vi "h.ACQ.GetFullSpectrumStreamToStoragePercentComplete.vi"(8 "error in":errorcluster, 11 "Connection ID":refnum<k5>) -> (0 "error out":errorcluster, 2 "Percent Complete":i32, 3 "Connection ID out":refnum<k5>)   [LabVIEW 2016, in "h.Library.lvlib"]
uses:
  h.Library.lvlib
panel:
  out "Content":u8[](array[numeric])
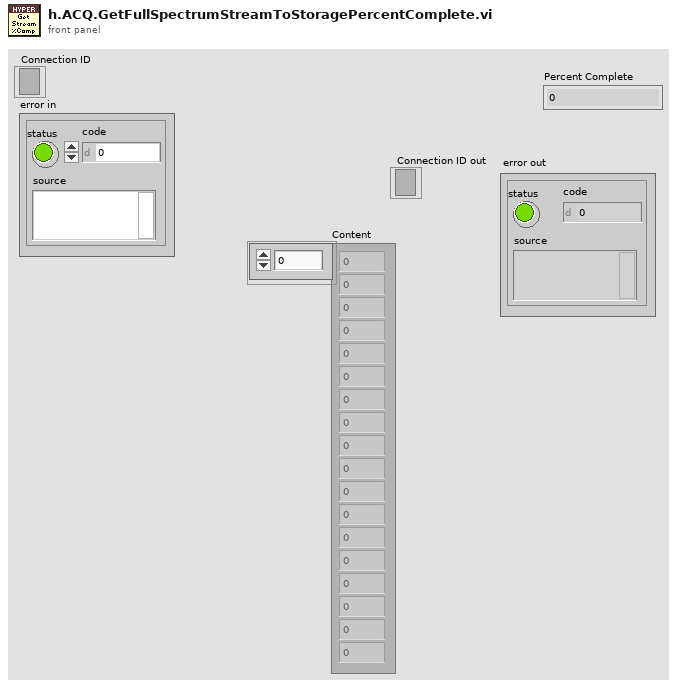
[diagram p1: front panel]
types:
  T1 = enum16{"big-endian, network order", "native, host order", "little-endian"}
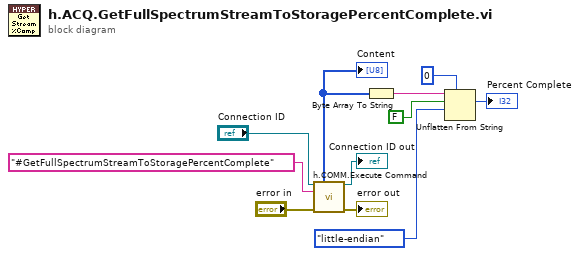
[diagram p0: block diagram]
diagram:
  n1 = call "h.COMM.Execute Command.vi"("Connection ID"="Connection ID", "Command"="#GetFullSpectrumStreamToStoragePercentComplete", "error in"="error in") -> ("Content"=w6:u8[], "Connection ID out"=→"Connection ID out":refnum<k5>, "error out"=→"error out":errorcluster)  [unwired: 5 in, 5 out]
  "Content" <- w6
  n2 = Byte Array To String(unsigned byte array=w6) -> (string=w5:string)
  n3 = Unflatten From String(type=0 ("laserscanspeed"), binary string=w5, data includes array or string size? (T)=FALSE, byte order (0:big-endian, network order)=T1."little-endian") -> (value=→"Percent Complete":i32)  [unwired: 1 in, 2 out]
